vi "On Selection Changed.vi"(7 "Action":T1, 11 "UI Data in":refnum<class "Settings UI.lvclass">) -> (3 "UI Data out":refnum<class "Settings UI.lvclass">)   [LabVIEW 2020, in "Output Sequencer.lvlib" / "Settings UI.lvclass"]
uses:
  Settings UI.lvclass
  Types/Settings UI Action.ctl
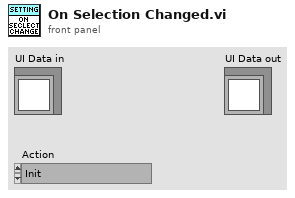
[diagram p1: front panel]
types:
  T1 = typedef "Output Sequencer.lvlib/Settings UI.lvclass/Settings UI Action.ctl" = enum16{"Init", "Timeout", "Tree Change", "Tree Mouse Down/Up", "Value Change", "Expand All", "Show Overview", "Collapse All", "Insert Above", "Insert Below", "Remove Step", "Move Up", "Move Down", "Drag Starting", "Drag Over", "Drop", "Drag Ended", "Import"}
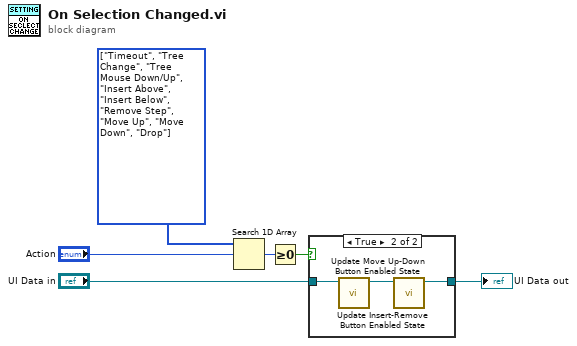
[diagram p0: block diagram]
diagram:
  w5 = T1[] [enum."Timeout", enum."Tree Change", enum."Tree Mouse Down/Up", enum."Insert Above", enum."Insert Below", enum."Remove Step", enum."Move Up", enum."Move Down", enum."Drop"] items=["Init", "Timeout", "Tree Change", "Tree Mouse Down/Up", "Value Change", "Expand All", "Show Overview", "Collapse All", "Insert Above", "Insert Below", "Remove Step", "Move Up", "Move Down", "Drag Starting", "Drag Over", "Drop", "Drag Ended", "Import"]
  n1 = Search 1D Array(1D array=w5, element="Action") -> (index of element=w4:i32)  [unwired: 1 in]
  n2 = Greater Or Equal To 0?(x=w4) -> (x >= 0?=w3:bool)
  n3 = case shown="True" w3 {
    tunnel: "UI Data in" -> [w7 w10]
    tunnel: [w7 w8] -> w1
    frame False {
    }
    frame True {
      n4 = call "Update Insert-Remove Button Enabled State.vi"("UI Data in"=w10) -> ("UI Data out"=w9:refnum<class "Settings UI.lvclass">)  [unwired: 10 in]
      n5 = call "Update Move Up-Down Button Enabled State.vi"("UI Data in"=w9) -> ("UI Data out"=w8:refnum<class "Settings UI.lvclass">)  [unwired: 10 in]
    }
  }
  "UI Data out" <- w1
